vi "read TBM configuration.vi"(8 "error in":errorcluster, 11 "Getting Started IO editor node in":refnum<class "UI Reference editor node.lvclass">) -> (0 "error out":errorcluster, 2 "configuration":refnum<class "TBM configuration.lvclass">, 3 "Getting Started IO editor node out":refnum<class "UI Reference editor node.lvclass">)   [LabVIEW 2013, in "UI Reference editor node.lvclass"]
uses:
  UI Reference editor node.lvclass
  <vilib>/NI/Tag Bus Module Framework/root configuration/TBM configuration.lvclass
  UI Reference editor node.lvclass/UI Reference editor node.ctl
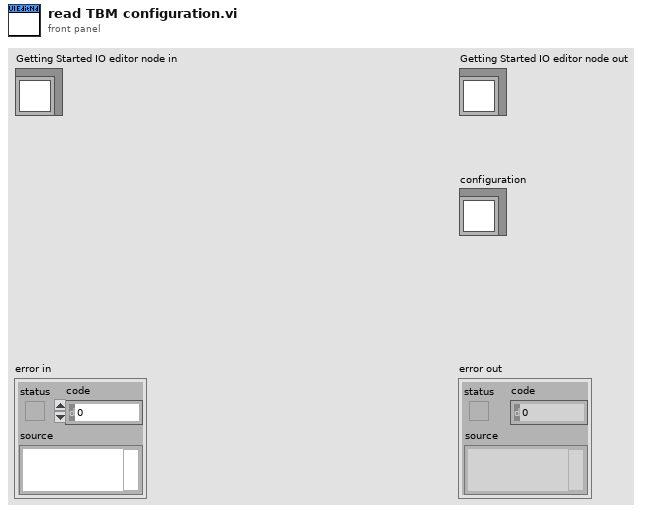
[diagram p1: front panel]
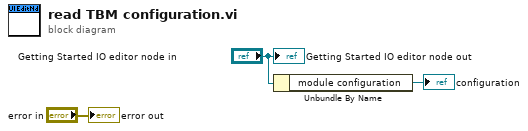
[diagram p0: block diagram]
diagram:
  n1 = Unbundle By Name("Getting Started IO editor node in") -> ("module configuration"=→"configuration":refnum<class "UI Reference configuration.lvclass">)
  "error out" <- "error in"
  "Getting Started IO editor node out" <- "Getting Started IO editor node in"
